vi "compare signals.vi"() -> ()   [LabVIEW 2018]
panel:
  in  "Average to use?":dbl
  in  "Data contains averages?":bool
  in  "Germanium Data":path=path "test.tdms" caption="Filename"
  out "Numeric":i32
  out "Ratio Between Scaled Diode Outputs":dbl[](graph)
  in  "poolarimeter map path":path=path "C:/Users/severinm/Box/Improving Constraints of Short-Range Spin-Dependent Forces/ARIADNE/He 3 polarization/Plasma Reigniter/Data/polarimeter map.lvm" caption="Filename"
  in  "germanium map path":path=path "C:/Users/severinm/Box/Improving Constraints of Short-Range Spin-Dependent Forces/ARIADNE/He 3 polarization/Plasma Reigniter/Data/germanium map.lvm" caption="Filename"
  in  "Polarimeter data":path=path "test.tdms" caption="Filename"
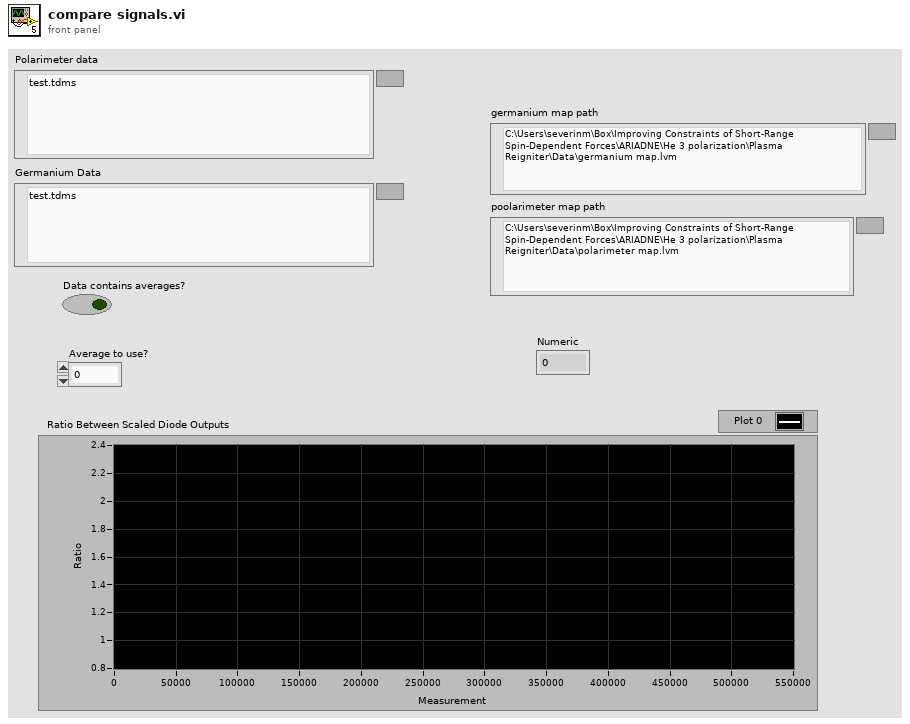
[diagram p1: front panel]
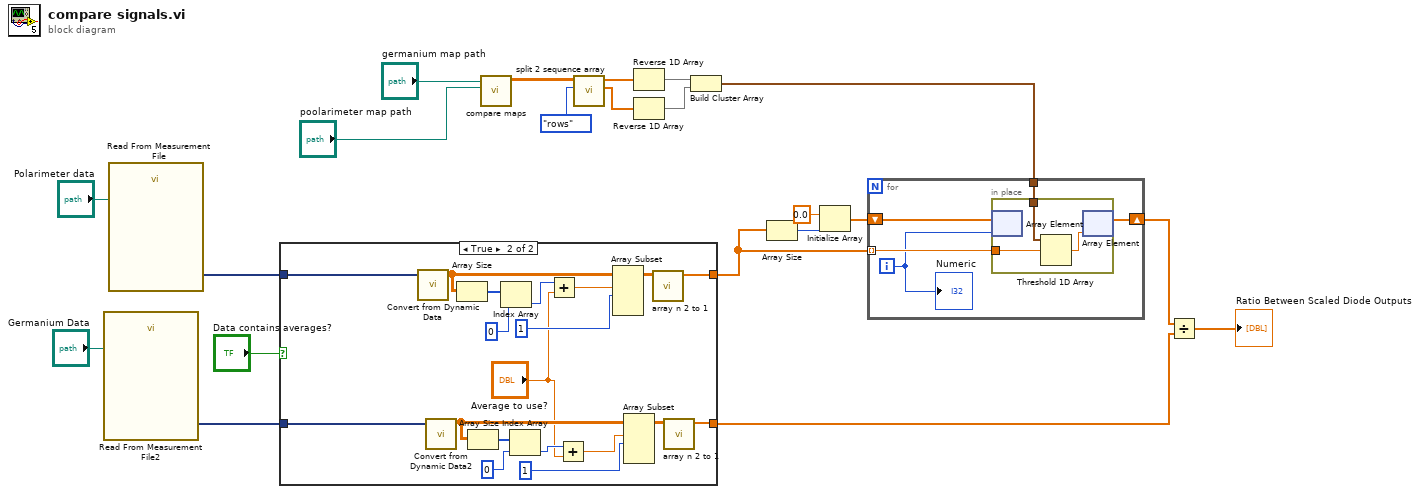
[diagram p0: block diagram]
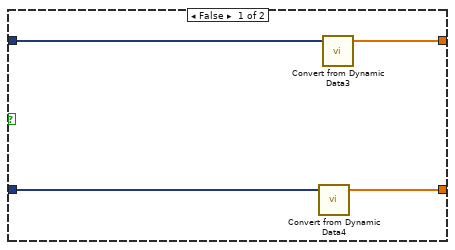
[diagram p2: hidden frame]
diagram:
  n1 = call "Read From Measurement File2"("Filename"="Germanium Data") -> ("Signals"=w11:dynamicdata)  [unwired: 5 in, 5 out]
  n2 = call "Read From Measurement File"("Filename"="Polarimeter data") -> ("Signals"=w15:dynamicdata)  [unwired: 5 in, 5 out]
  n3 = case shown="True" "Data contains averages?" {
    tunnel: w15 -> [w23 w44]
    tunnel: [w22 w39] -> w1
    tunnel: w11 -> [w25 w43]
    tunnel: [w24 w36] -> w10
    frame False {
      n4 = call "Convert from Dynamic Data4"("Dynamic Data Type"=w25) -> ("Array"=w24:dbl[])  [unwired: 3 in]
      n5 = call "Convert from Dynamic Data3"("Dynamic Data Type"=w23) -> ("Array"=w22:dbl[])  [unwired: 3 in]
    }
    frame True {
      n6 = call "Convert from Dynamic Data"("Dynamic Data Type"=w44) -> ("Array"=w42:dbl[][])  [unwired: 3 in]
      n7 = call "Convert from Dynamic Data2"("Dynamic Data Type"=w43) -> ("Array"=w35:dbl[][])  [unwired: 3 in]
      n8 = Array Size(array=w42) -> (size(s)=w41:i32[])
      n9 = Array Size(array=w35) -> (size(s)=w38:i32[])
      n10 = Index Array(array=w41, index=0) -> (element=w28:i32)
      n11 = Index Array(array=w38, index=0) -> (element=w27:i32)
      n12 = Add(x=w28, y="Average to use?") -> (x+y=w30:dbl)
      n13 = Add(x=w27, y="Average to use?") -> (x+y=w29:dbl)
      n14 = Array Subset(array=w42, index (row)=w30, length (row)=1 ("index")) -> (w40:dbl[][])  [unwired: 2 in]
      n15 = Array Subset(array=w35, index (row)=w29, length (row)=1 ("index")) -> (w37:dbl[][])  [unwired: 2 in]
      n16 = call "array n 2 to 1.vi"("2N array"=w40) -> ("1N array"=w39:dbl[])  [unwired: 10 in]
      n17 = call "array n 2 to 1.vi"("2N array"=w37) -> ("1N array"=w36:dbl[])  [unwired: 10 in]
    }
  }
  n18 = call "compare maps.vi"("poolarimeter map path"="poolarimeter map path", "germanium map path"="germanium map path") -> ("germainium to polarimeter map"=w19:dbl[][])  [unwired: 9 in]
  n19 = call "split 2 sequence array.vi"("Enum"=enum16{"columns", "rows"}."rows", "2 sequence array"=w19) -> ("i1 sequence"=w17:dbl[], "i0 sequence"=w16:dbl[])  [unwired: 8 in]
  n20 = Reverse 1D Array(array=w16) -> (reversed array=w9:dbl[])
  n21 = Reverse 1D Array(array=w17) -> (reversed array=w8:dbl[])
  n22 = Build Cluster Array(w9, w8) -> (w13:cluster{dbl, dbl}[])
  n23 = Array Size(array=w1) -> (size(s)=w3:i32)
  n24 = Initialize Array(0.0 ("element"), w3) -> (w2:dbl[])
  n25 = for {
    tunnel: w1 -> [w48] mode=indexing
    tunnel: w13 -> [w49]
    shift-right: [w45] -> w6
    shift-left: w2 -> [w46]
    i -> [w47]
    n26 = in-place {
      in-place-border: w49 -> [w52]
      in-place-border: w48 -> [w51]
      n27 = in-place-array #1(w46, w47) -> ()  [unwired: 1 out]
      n28 = Threshold 1D Array(2:w51, 3:w52) -> (0:w50:dbl)  [unwired: 1 in]
      n29 = in-place-array #1(w50) -> (w45:dbl[])  [unwired: 1 out]
    }
    "Numeric" <- w47
  }
  n30 = Divide(x=w6, y=w10) -> (x/y=→"Ratio Between Scaled Diode Outputs":dbl[])
